vi "Date format to text sortable.vi"(8 "error in (no error)":errorcluster, 11 "Date time string":string) -> (0 "error out":errorcluster, 3 "New date time string":string)   [LabVIEW 2013]
panel:
  out "seconds":string
  out "PM?":bool
  out "minute":string
  out "hour":string
  out "year":string
  out "day":string="Day"
  out "month":string
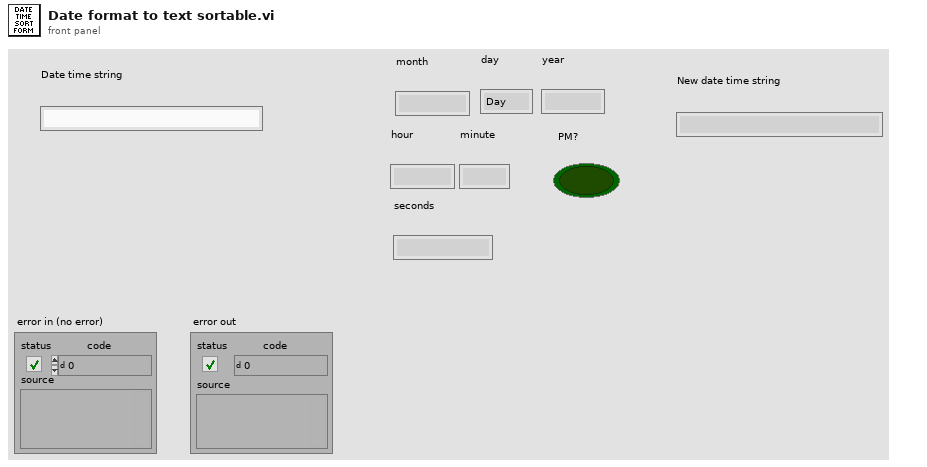
[diagram p1: front panel]
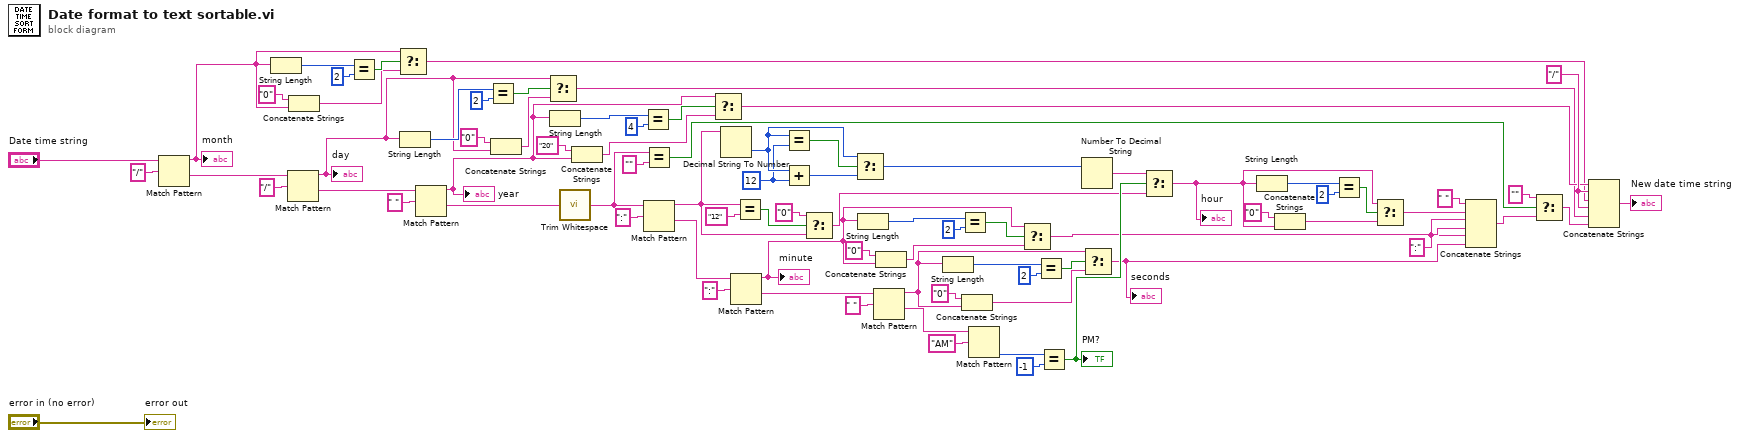
[diagram p0: block diagram]
diagram:
  w36 = 12 ("y")
  w8 = ":" ("string")
  w57 = "/" ("string")
  n1 = Match Pattern(string="Date time string", regular expression="/") -> (before substring=w66:string, after substring=w79:string)  [unwired: 1 in, 2 out]
  "month" <- w66
  n2 = String Length(string=w66) -> (length=w69:i32)
  n3 = Match Pattern(string=w79, regular expression="/") -> (before substring=w58:string, after substring=w77:string)  [unwired: 1 in, 2 out]
  "day" <- w58
  n4 = Concatenate Strings("0" ("string"), w66) -> (w64:string)
  n5 = Equal?(x=w69, y=2) -> (x = y?=w67:bool)
  n6 = Select(t=w66, s=w67, f=w64) -> (s? t:f=w25:string)
  n7 = String Length(string=w58) -> (length=w59:i32)
  n8 = Match Pattern(string=w77, regular expression=" ") -> (before substring=w51:string, after substring=w71:string)  [unwired: 1 in, 2 out]
  "year" <- w51
  n9 = Equal?(x=w59, y=2) -> (x = y?=w61:bool)
  n10 = Concatenate Strings("0" ("string"), w58) -> (w63:string)
  n11 = Select(t=w58, s=w61, f=w63) -> (s? t:f=w24:string)
  n12 = String Length(string=w51) -> (length=w56:i32)
  n13 = call <vilib>:"Trim Whitespace.vi"("string"=w71) -> ("trimmed string"=w6:string)  [unwired: 1 in]
  n14 = Concatenate Strings("20" ("string"), w51) -> (w52:string)
  n15 = Equal?(x=w56, y=4) -> (x = y?=w54:bool)
  n16 = Equal?(x=w6, y="") -> (x = y?=w4:bool)
  n17 = Match Pattern(string=w6, regular expression=":") -> (before substring=w28:string, after substring=w18:string)  [unwired: 1 in, 2 out]
  n18 = Select(t=w51, s=w54, f=w52) -> (s? t:f=w26:string)
  n19 = Decimal String To Number(string=w28) -> (number=w37:i32)  [unwired: 2 in, 1 out]
  n20 = Match Pattern(string=w18, regular expression=":") -> (before substring=w22:string, after substring=w21:string)  [unwired: 1 in, 2 out]
  "minute" <- w22
  n21 = Equal?(x=w28, y="12") -> (x = y?=w30:bool)
  n22 = Equal?(x=w37, y=w36) -> (x = y?=w38:bool)
  n23 = Add(x=w37, y=w36) -> (x+y=w35:i32)
  n24 = Select(t="0", s=w30, f=w28) -> (s? t:f=w27:string)
  n25 = Select(t=w37, s=w38, f=w35) -> (s? t:f=w34:i32)
  n26 = String Length(string=w22) -> (length=w45:i32)
  n27 = Match Pattern(string=w21, regular expression=" ") -> (before substring=w13:string, after substring=w19:string)  [unwired: 1 in, 2 out]
  n28 = Concatenate Strings("0" ("string"), w22) -> (w41:string)
  n29 = String Length(string=w13) -> (length=w16:i32)
  n30 = Equal?(x=w45, y=2) -> (x = y?=w43:bool)
  n31 = Concatenate Strings("0" ("string"), w13) -> (w14:string)
  n32 = Match Pattern(string=w19, regular expression="AM") -> (offset past match=w73:i32)  [unwired: 1 in, 3 out]
  n33 = Select(t=w22, s=w43, f=w41) -> (s? t:f=w9:string)
  n34 = Equal?(x=w16, y=2) -> (x = y?=w15:bool)
  n35 = Equal?(x=w73, y=-1) -> (x = y?=w39:bool)
  "PM?" <- w39
  n36 = Number To Decimal String(number=w34) -> (decimal integer string=w33:string)  [unwired: 1 in]
  n37 = Select(t=w13, s=w15, f=w14) -> (s? t:f=w7:string)
  "seconds" <- w7
  n38 = Select(t=w33, s=w39, f=w27) -> (s? t:f=w32:string)
  "hour" <- w32
  n39 = String Length(string=w32) -> (length=w46:i32)
  n40 = Concatenate Strings("0" ("string"), w32) -> (w50:string)
  n41 = Equal?(x=w46, y=2) -> (x = y?=w48:bool)
  n42 = Select(t=w32, s=w48, f=w50) -> (s? t:f=w10:string)
  n43 = Concatenate Strings(" " ("string"), w10, w8, w9, w8, w7) -> (w2:string)
  n44 = Select(t="", s=w4, f=w2) -> (s? t:f=w1:string)
  n45 = Concatenate Strings(w26, w57, w25, w57, w24, w1) -> (→"New date time string":string)
  "error out" <- "error in (no error)"
